vi "Finish.vi"   [LabVIEW 2023]
doc: "This VI is called during exit. It can be used to close I/O refnums, save collected data, etc."
uses:
  <vilib>/Rock Robotics/WPI/ThirdParty/REV Robotics/REVLib/Typedef/Spark MAX Control Type.ctl
  <vilib>/Rock Robotics/WPI/Utilities/WPI_GetSetVariantRefNum.vi
types:
  T1 = typedef "WPI_JoystickDevRef.ctl" = cluster{"Device":T2}
  T2 = typedef "WPI_JoystickDeviceEnum.ctl" = enum16{"USB 0", "USB 1", "USB 2", "USB 3", "USB 4", "USB 5"}
  T3 = typedef "WPI_MotorControlDeviceRef.ctl" = cluster{"DeviceStatus":errorcluster, "Type":T4, "PWM":cluster{"PWM Channel":T5, "DeadBand":T6}, "CAN":cluster{"Device Number":u8, "SetOutput VI Ref":variant, "GetOutput VI Ref":variant, "Enable VI Ref":variant, "Disable VI Ref":variant, "Data":variant}, "Invert":bool, "DIO PWM":cluster{"PWM \"Enable\" Channel":T5, "DIOChannel":T7, "PWM Rate":dbl}}
  T4 = typedef "WPI_MotorControlType.ctl" = enum16{"PWM", "CAN", "DIO PWM"}
  T5 = typedef "FPGA_DIOPWMChannel.ctl" = enum8{"PWM 0", "PWM 1", "PWM 2", "PWM 3", "PWM 4", "PWM 5", "PWM 6", "PWM 7", "PWM 8", "PWM 9", "PWM MXP 0", "PWM MXP 1", "PWM MXP 2", "PWM MXP 3", "PWM MXP 4", "PWM MXP 5", "PWM MXP 6", "PWM MXP 7", "PWM MXP 8", "PWM MXP 9", "Invalid"}
  T6 = typedef "WPI_PWMDeadband.ctl" = cluster{"Name":string, "maxPositivePwm":i32, "minPositivePwm":i32, "centerPwm":i32, "maxNegativePwm":i32, "minNegativePwm":i32, "angularRange":u16}
  T7 = typedef "FPGA_DIOChannel.ctl" = enum8{"DIO 0", "DIO 1", "DIO 2", "DIO 3", "DIO 4", "DIO 5", "DIO 6", "DIO 7", "DIO 8", "DIO 9", "DIO MXP 0", "DIO MXP 1", "DIO MXP 2", "DIO MXP 3", "DIO MXP 4", "DIO MXP 5", "DIO MXP 6", "DIO MXP 7", "DIO MXP 8", "DIO MXP 9", "DIO MXP 10", "DIO MXP 11", "DIO MXP 12", "DIO MXP 13", "DIO MXP 14", "DIO MXP 15", "SPI Port CS1", "SPI Port CS2", "SPI Port CS3", "SPI Port MISO", "SPI Port MOSI", "Invalid"}
  T8 = typedef "Spark MAX Control Type.ctl" = enum16{"Percent VBus", "Voltage", "Velocity", "Position", "Smart Motion", "Current", "Smart Velocity"}
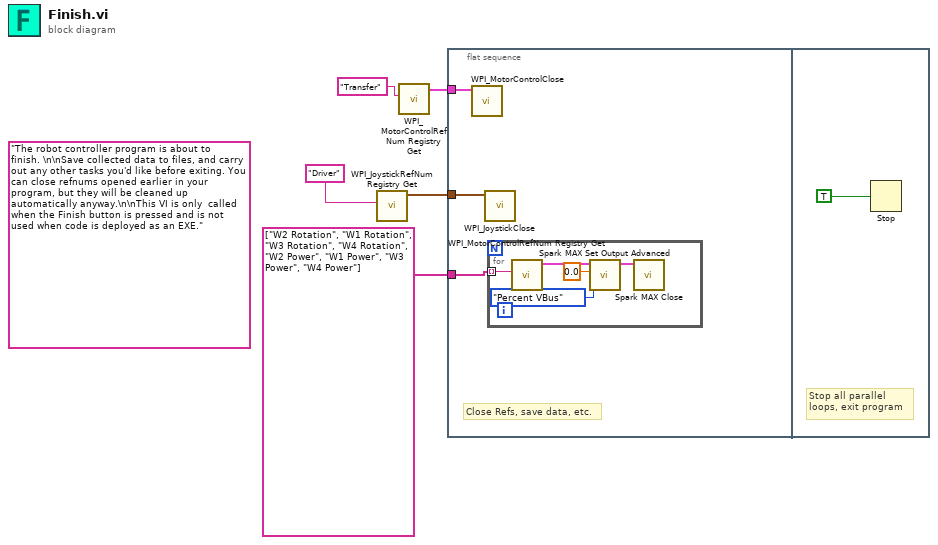
[diagram p0: block diagram]
diagram:
  (unwired) "The robot controller program is about to finish. \n\nSave collected data to files, and carry out any other tasks you'd like before exiting. You can close refnums opened earlier in your program, but they will be cleaned up automatically anyway.\n\nThis VI is only  called when the Finish button is pressed and is not used when code is deployed as an EXE."
  n1 = call <vilib>:"WPI_JoystickRefNum Registry Get.vi"("refnum name"="Driver") -> ("JoystickDevRef"=w4:T1)  [unwired: 1 in, 9 out]
  n2 = call <vilib>:"WPI_MotorControlRefNum Registry Get.vi"("refnum name"="Transfer") -> ("MotorControlDevRef"=w1:T3)  [unwired: 9 in, 1 out]
  n3 = flat-sequence {
    tunnel: w4 -> [w8]
    tunnel: string[] ["W2 Rotation", "W1 Rotation", "W3 Rotation", "W4 Rotation", "W2 Power", "W1 Power", "W3 Power", "W4 Power"] ("refnum name") -> [w7]
    tunnel: w1 -> [w6]
    frame #0 {
      # "Close Refs, save data, etc."
      n4 = call <vilib>:"WPI_MotorControlClose.vi"("MotorControlDevRef"=w6) -> ()  [unwired: 10 in, 1 out]
      n5 = call <vilib>:"WPI_JoystickClose.vi"("JoystickDevRef"=w8) -> ()  [unwired: 11 out]
      n6 = for {
        tunnel: w7 -> [w13] mode=indexing
        n7 = call <vilib>:"WPI_MotorControlRefNum Registry Get.vi"("refnum name"=w13) -> ("MotorControlDevRef"=w12:T3)  [unwired: 9 in, 1 out]
        n8 = call <vilib>:"Spark MAX Set Output Advanced.vi"("Control Mode"=Spark_MAX_Control_Type."Percent VBus", "Setpoint"=0.0, "MotorControlDevRef"=w12) -> ("MotorControlDevRef"=w11:T3)  [unwired: 7 in, 1 out]
        n9 = call <vilib>:"Spark MAX Close.vi"("MotorControlDeviceRef"=w11) -> ()  [unwired: 10 in, 1 out]
      }
    }
    frame #1 {
      # "Stop all parallel\nloops, exit program"
      n10 = Stop(stop? (T)=TRUE ("Quit")) -> ()
    }
  }
